vi "BRig_dataMTrig_warmup_cNoLick_R.vi"() -> (2 "output_warmup_cNoLick_R":i32)   [LabVIEW 2014]
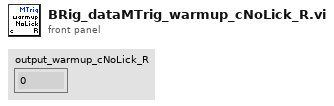
[diagram p1: front panel]
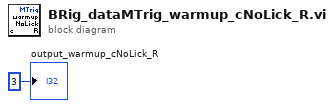
[diagram p0: block diagram]
diagram:
  "output_warmup_cNoLick_R" <- 3 ("output_iBlock")
